vi "Test PC from CnfgFile.vi"() -> ()   [LabVIEW 2009, in "POLARIS BME DG.lvlib"]
doc: "This VI is a example for usage of POLARIS BME DG.lvlib classes.\n\nUSAGE:\n1. Select Your .bmedg configiration file, with has been created with Configure Systems.vi\n2. Select directory that contains calibration filesl Modules.cal and BME_G0x.cal\n3. Enter the name of the system whose channels Your want to modify\n4. Run VI\n5. Update Chnl Direct writes channel settings into HW with immediately deactivation, modify and activation of all system DGs. This will cause a common shot at all channels after activation. Please keep it in mind, if Your plant needs some pause between tho following shots e.g. for cool down.\n\n6. UpdateChnl synchron use mechanism of DG type SG08P2. You need to configure cards and channels properly for this reasen. All cards must have the same MS-Bus configuration and Bit \"LoadDataOnBus = 0x80\" mus be set. If all output modulo couner reach zero at MASTERCARD, mastercard puts a signal to slavecard to load new parameters.\n\n7. \"Update Chnl wait\" can be used if channels have slow repetition rate compared with polling rate of ReadTriggerCounter. Programm wait close before next common shot would fall and updates parameter with de and reactivate of all cards.\n\nIMPLEMENTATION: See comments in blockdiagramm.\n\n\n-----------------\n\nauthor: Alexander Kessler, Helmholtz-Institut-Jena \nmaintainer: Alexander Kessler: alexander.kessler@uni-jena.de\n\nLicense Agreement for this software:\n\nCopyright (C)\nHelmholtz-Institut-Jena\nFröbelsteg 3\n07743 Jena\nGermany\n\nContact: alexander.kessler@uni-jena.de\n\nThis program is free software; you can redistribute it and/or modify it under the terms of the GNU General Public License as published by the Free Software Foundation; either version 2 of the license, or (at your option) any later version.\n\nThis program is distributed in the hope that it will be useful, but WITHOUT ANY WARRANTY; without even the implied warranty of MERCHANTABILITY or FITNESS FOR A PARTICULAR PURPOSE. See the GNU General License for more details (http://www.gnu.org)."
uses:
  POLARIS BME DG.lvlib
  LV-BME Interface/ChnlSettings.ctl
  LV-BME Interface/Chnl Settings Complete.ctl
  LV-BME Interface/Go_Done_Chnl_Settings.ctl
  LV-BME Interface/GoSignalBits.ctl
  LV-BME Interface/SG08_Chnl_Settings.ctl
  DG Classes/BME_DG_Chnl/BME_DG_Chnl.lvclass
  DG Classes/BME_DG_Base/BME_DG_Base.lvclass
  DG Classes/BME_DG_System/BME_DG_System.lvclass
panel:
  out "ChnlPeriods":dbl[][](array[numeric])
  in  "Save Changes":bool=TRUE
  out "Master Trigger Counter":i64
  in  "SystemlName":u16(ring) items=["MiraSync", "MS"]
  in  "UpdateChnl Synchron":bool=TRUE
  in  "ChnlParam":T1={"Channel Name"="", "ChnParameter"={" Delay (µs)"=0.0, "On?"=FALSE, "PositiveVoltage?"=TRUE, "50OhmTerminated? "=FALSE, "25OhmOutput?"=FALSE}, "DelayFormula"="", "OutputModulo"=1, "Go and Done Signal"={"Go Signal"=16, "Done Signal"=16}, "G08_Chnl_Settings"={"Pulse Width (µs)"=0.1, "Output Offset"=0, "Disconnect (E,F)"=FALSE, "Onto MsBus (E,F)"=FALSE, "Input Positive (E,F)"=TRUE}} {"ChnParameter"."Delay (µs)" min=0.0 max=100000000.0 format="%.4f"; "G08_Chnl_Settings"."Pulse Width (µs)" min=0.0 max=8947840.0 format="%#.6f"; "Go and Done Signal"."Done Signal" format="%04x" items=["Local Primary"=1, "Local Secondary"=2, "Local Force"=4, "Master Primary"=16]; "Go and Done Signal"."Go Signal" format="%04x" items=["Local Primary0x1"=1, "Local Secondary0x2"=2, "Local Force 0x4"=4, "Resynchronize 0x8"=8, "Master Prim. 0x10"=16, "Master Sec. 0x20"=32, "Master Force  0x40"=64, "System Clock 0x80"=128, "Delay Clock 0x100"=256, "Inhibit Local 0x200"=512, "Start Local 0x400"=1024, "Start Bus 0x800"=2048, "Step Back Local 0x1000"=4096, "Step Back Bus 0x2000"=8192, "RunCircle 0x4000"=16384, "SyncReload 0x8000"=32768, "From E 0x10000"=65536, "From F 0x20000"=131072, "From Bus 0x40000"=262144]}
  in  "Update Chnl direct":bool=TRUE
  in  "pathCalFilesDir":path=path "C:/CS Framework/pwpc74-Config"
  in  "pathConfigFile":path=path "C:/CS Framework/pwpc74-Config/pwpc74.bmedg"
  out "Problem Chnls out":string[](array[string])
  in  "Reset Error":bool
  out "error out":errorcluster
  in  "Update Delay direct":bool=TRUE
  in  "UpdateChnl wait":bool=TRUE
  in  "ChnlParameter":T6 {"ChnParam2write"."Delay (µs)" min=0.0 max=100000000.0 format="%.4f"}
  out "Counts till common shot":i32=2147483647
  out "Interrupts":u32[](array[numeric])=[11153, 10240, 10240, 10240, 11008, 11008, 10240, 10240, 10240] format="%b"
  in  "stop 2":bool=TRUE
  in  "ReadStatus":bool=TRUE
  in  "Activate Card":bool=TRUE
  in  "ResetModuloCounters":bool=TRUE
  in  "Selected Chnl":u16(ring) items=["TrigDelay", "A1LDD", "A3LDD", "A4LDD", "A5LDD", "Reserve", "PulsP On", "PulsP Off", "A1 PC On", "A1 PC Off", "Oszi", "Kamera"]
  in  "Card":u16(ring) items=["Master", "Slave1"]
  in  "STOP":bool
  # "ATTENTION, WORKS ONLY\nif a MASTER CHNL  is set to \nsync update!!! Otherwise undefined\nDelay states occur."
  # "Calls of DLL \nSet_G08_Delay\nhave no effect\nindependent of sync\nsettings\n201207-10\n\n201211-26 LoadCardParam\ncall is needed"
  # "Funktioniert nicht, das Problem liegt daran, dass ulong ReadInterruptStatus(long DG_Number) die Interruptbits nicht\nzuverlässig ausliest."
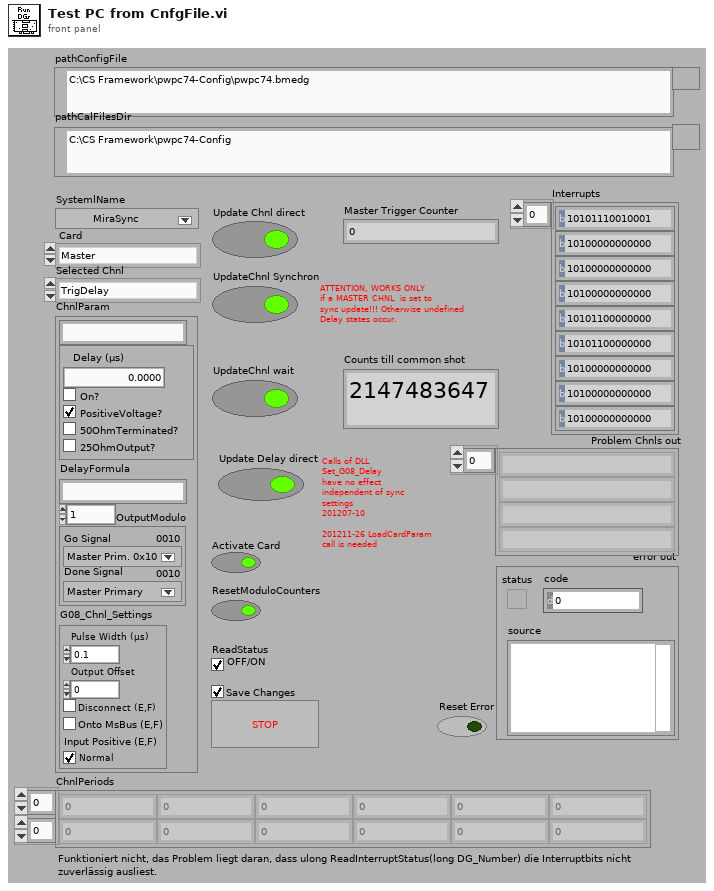
[diagram p1: front panel]
types:
  T1 = typedef "POLARIS BME DG.lvlib/Chnl Settings Complete.ctl" = cluster{"Channel Name":string, "ChnParameter":T2, "DelayFormula":string, "OutputModulo":i32, "Go and Done Signal":T3, "G08_Chnl_Settings":T5}
  T2 = typedef "POLARIS BME DG.lvlib/ChnlSettings.ctl" = cluster{" Delay (µs)":dbl, "On?":bool, "PositiveVoltage?":bool, "50OhmTerminated? ":bool, "25OhmOutput?":bool}
  T3 = typedef "POLARIS BME DG.lvlib/Go_Done_Chnl_Settings.ctl" = cluster{"Go Signal":T4, "Done Signal":u32}
  T4 = typedef "POLARIS BME DG.lvlib/GoSignalBits.ctl" = u32
  T5 = typedef "POLARIS BME DG.lvlib/SG08_Chnl_Settings.ctl" = cluster{"Pulse Width (µs)":dbl, "Output Offset":u32, "Disconnect (E,F)":bool, "Onto MsBus (E,F)":bool, "Input Positive (E,F)":bool}
  T6 = cluster{"ChnlName":string, "ChnParam2write":T2, "TriggerModulo":u32}
  T7 = enum16{"GetSystem", "SetSystem", "FirstInit", "ForceInit", "Release"}
  T8 = enum8{"Enabled", "Disabled", "Disabled and Grayed Out"}
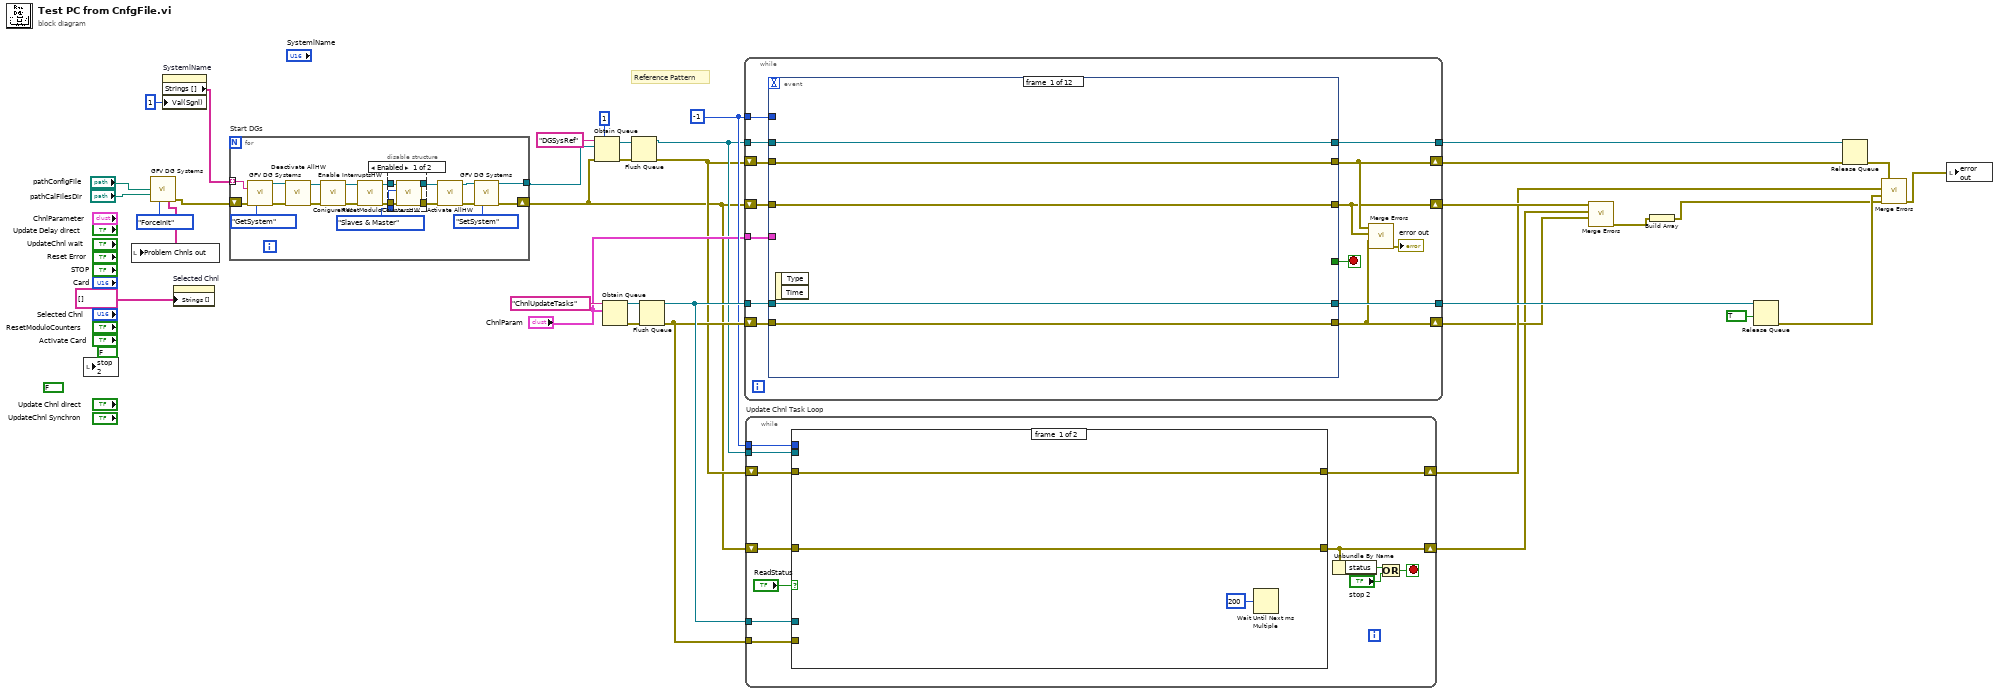
[diagram p0: block diagram]
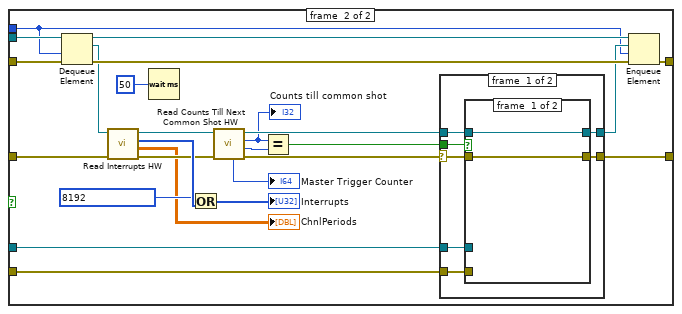
[diagram p3: hidden frame]
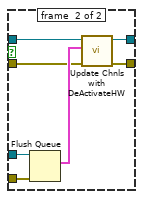
[diagram p4: hidden frame]
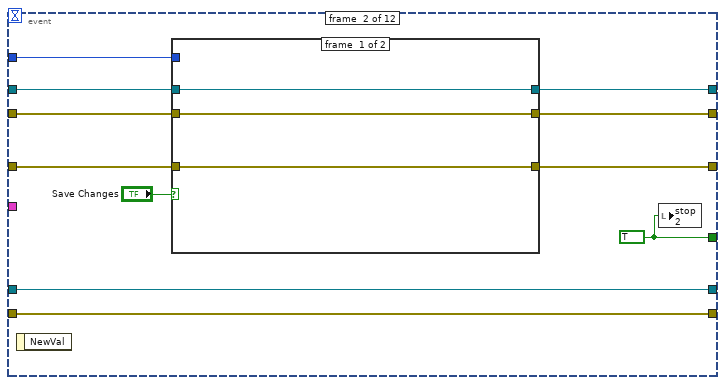
[diagram p6: hidden frame]
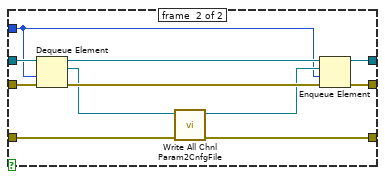
[diagram p7: hidden frame]
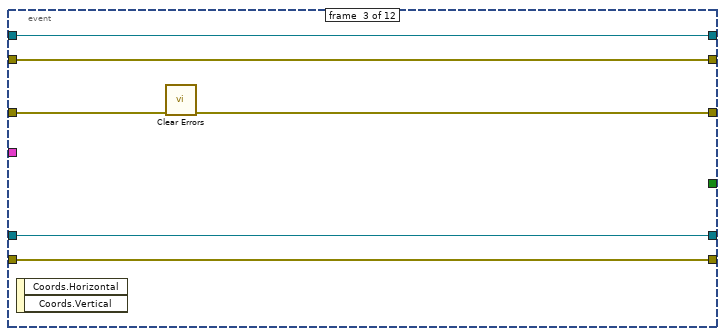
[diagram p8: hidden frame]
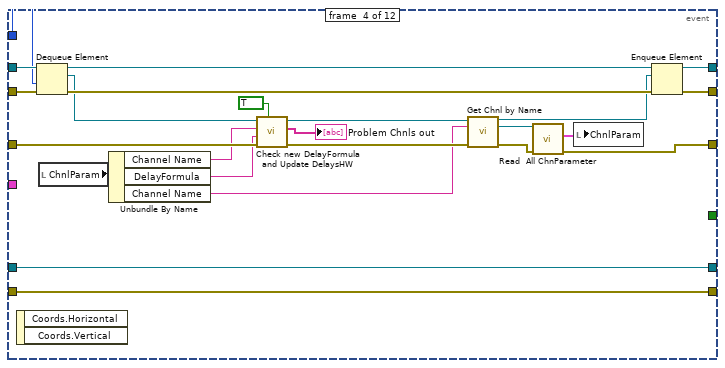
[diagram p9: hidden frame]
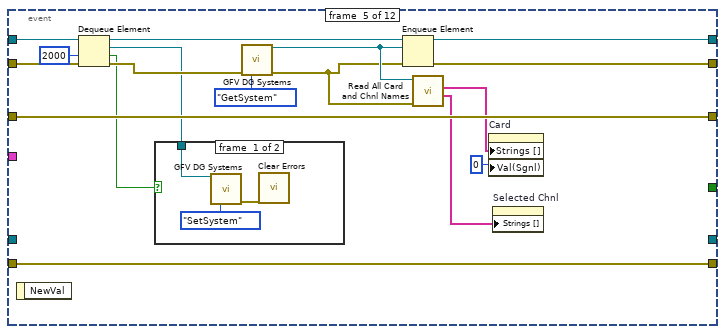
[diagram p10: hidden frame]
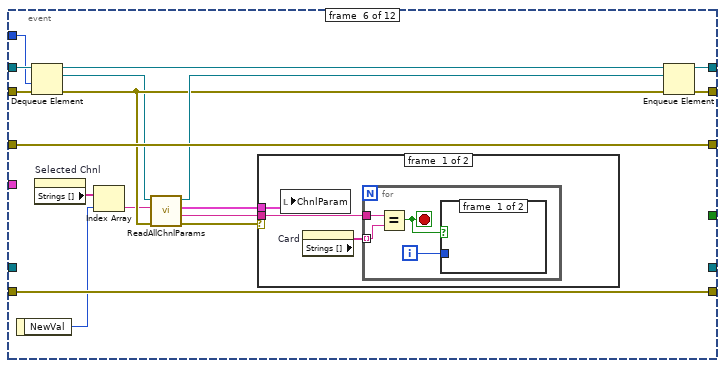
[diagram p12: hidden frame]
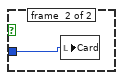
[diagram p13: hidden frame]
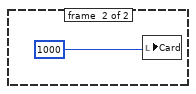
[diagram p14: hidden frame]
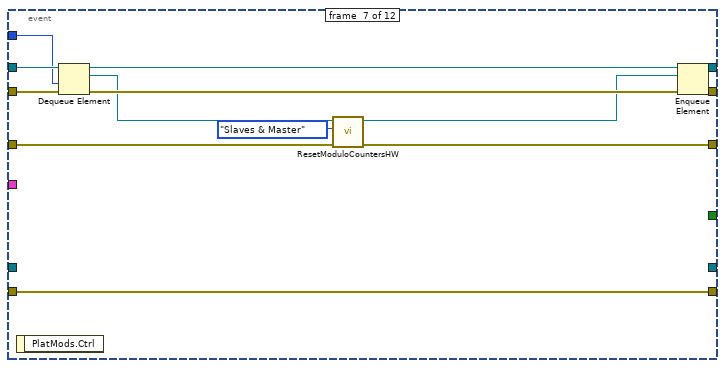
[diagram p15: hidden frame]
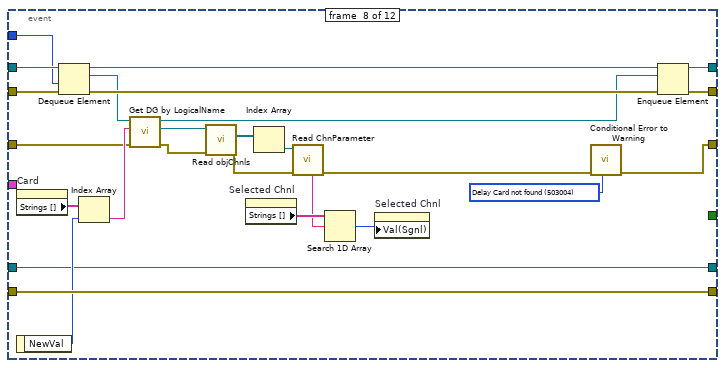
[diagram p16: hidden frame]
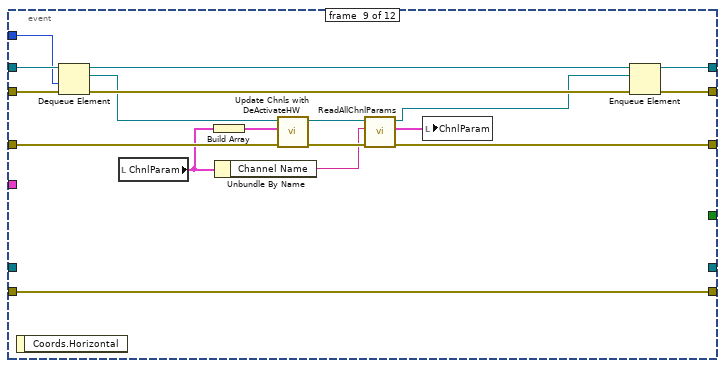
[diagram p17: hidden frame]
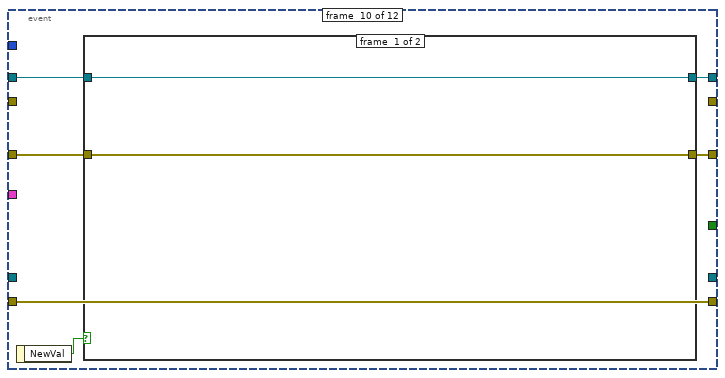
[diagram p18: hidden frame]
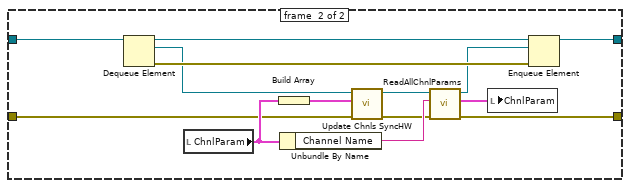
[diagram p19: hidden frame]
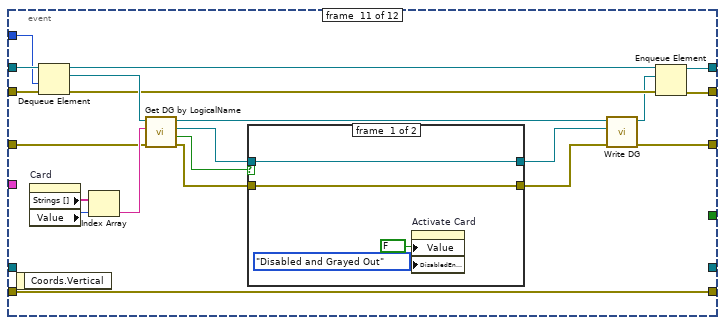
[diagram p20: hidden frame]
diagram:
  w23 = -1 ("timeout in ms (-1)")
  (unwired) FALSE ("stop 3")
  # "Reference Pattern"
  n1 = local write "stop 2"(FALSE ("stop 2")) -> ()
  n2 = call "GFV DG Systems.vi"("Config File"="pathConfigFile", "Dir Calibration files"="pathCalFilesDir", "Mode"=T7."ForceInit") -> ("Problem Chnls out"=w13:string[], "error out"=w14:errorcluster)  [unwired: 7 in, 4 out]
  n3 = local write "Problem Chnls out"(w13) -> ()
  n4 = property on="SystemlName" class="Ring (strict)"("Val(Sgnl)"=u16 1 ("Value (Signaling)")) -> ("Strings []"=w12:string[])  [unwired: 2 in, 2 out]
  n5 = property on="Selected Chnl" class="Ring (strict)"("Strings []"=string[] []) -> ()  [unwired: 2 in, 2 out]
  n6 = for "Start DGs" {
    shift-right: [w39] -> w8
    shift-left: w14 -> [w45]
    tunnel: w12 -> [w44] mode=indexing
    tunnel: [w38] -> w7
    n7 = call "GFV DG Systems.vi"("SystemlName"=w44, "error in"=w45, "Mode"=T7."GetSystem") -> ("BME_DG_System out"=w43:refnum<class "BME_DG_System.lvclass">, "error out"=w46:errorcluster)  [unwired: 7 in, 4 out]
    n8 = call "Deactivate AllHW.vi"("error in (no error)"=w46, "BME_DG_System in"=w43) -> ("error out"=w55:errorcluster, "BME_DG_System out"=w56:refnum<class "BME_DG_System.lvclass">)  [unwired: 8 in]
    n9 = call "ConigureHW.vi"("error in (no error)"=w55, "BME_DG_System in"=w56) -> ("error out"=w53:errorcluster, "BME_DG_System out"=w54:refnum<class "BME_DG_System.lvclass">)  [unwired: 8 in]
    n10 = call "Enable InterruptsHW.vi"("error in (no error)"=w53, "BME_DG_System in"=w54) -> ("error out"=w50:errorcluster, "BME_DG_System out"=w51:refnum<class "BME_DG_System.lvclass">)  [unwired: 8 in]
    n11 = disable-structure shown="Enabled" {
      disable-tunnel: w51 -> [w61 w63]
      disable-tunnel: [w60 w63] -> w49
      disable-tunnel: w50 -> [w59 w62]
      disable-tunnel: [w58 w62] -> w48
      disable-tunnel: enum16{"Slaves only", "Slaves & Master"}."Slaves & Master" ("Enum") -> [w57 _]
      frame #0 {
        n12 = call "ResetModuloCountersHW.vi"("error in (no error)"=w59, "Enum"=w57, "BME_DG_System in"=w61) -> ("error out"=w58:errorcluster, "BME_DG_System out"=w60:refnum<class "BME_DG_System.lvclass">)  [unwired: 7 in]
      }
      frame #1 {
      }
    }
    n13 = call "Activate AllHW.vi"("error in (no error)"=w48, "BME_DG_System in"=w49) -> ("error out"=w41:errorcluster, "BME_DG_System out"=w42:refnum<class "BME_DG_System.lvclass">)  [unwired: 8 in]
    n14 = call "GFV DG Systems.vi"("BME_DG_System"=w42, "error in"=w41, "Mode"=T7."SetSystem") -> ("BME_DG_System out"=w38:refnum<class "BME_DG_System.lvclass">, "error out"=w39:errorcluster)  [unwired: 7 in, 4 out]
  }
  n15 = Obtain Queue(max queue size (-1, unlimited)=1, name (unnamed)="DGSysRef", element data type=w7, error in (no error)=w8) -> (queue out=w33:refnum<queue>, error out=w32:errorcluster)  [unwired: 1 in, 1 out]
  n16 = Obtain Queue(name (unnamed)="ChnlUpdateTasks", element data type="ChnlParam") -> (queue out=w28:refnum<queue>, error out=w29:errorcluster)  [unwired: 3 in, 1 out]
  n17 = Flush Queue(queue=w33, error in (no error)=w32) -> (queue out=w10:refnum<queue>, error out=w9:errorcluster)  [unwired: 1 out]
  n18 = Flush Queue(queue=w28, error in (no error)=w29) -> (queue out=w25:refnum<queue>, error out=w24:errorcluster)  [unwired: 1 out]
  n19 = while {
    shift-right: [w66] -> w21
    shift-left: w8 -> [w75]
    shift-right: [w67] -> w6
    shift-left: w9 -> [w73]
    tunnel: w10 -> [w76]
    tunnel: [w74] -> w34
    tunnel: w25 -> [w72]
    tunnel: "ChnlParam" -> [w71]
    tunnel: [w69] -> w27
    shift-right: [w65] -> w19
    shift-left: w24 -> [w70]
    tunnel: w23 -> [w68]
    stop <- w77 stop-if-true
    n20 = event shown="[1] \"STOP\": Value Change" {
      selector: _ -> [_ _ _ _ _ _ _ _ _ _ _ _]
      dyn-events: _ -> [_ _ _ _ _ _ _ _ _ _ _ _]
      timeout: _ -> [_ _ _ _ _ _ _ _ _ _ _ _]
      tunnel: [_ w83 _ _ _ _ _ _ _ _ _ _] -> w77
      tunnel: w76 -> [w82 w90 w112 w136 w152 w169 w196 w222 w240 w244 w272 w312]
      tunnel: w75 -> [w81 w89 w113 w128 w154 w174 w186 w209 w232 w242 w280 w311]
      tunnel: [w82 w86 w112 w132 w149 w167 w191 w217 w235 w243 w266 w312] -> w74
      tunnel: [w81 w84 w108 w116 w154 w174 w187 w199 w226 w241 w273 w311] -> w66
      tunnel: w73 -> [w80 w88 w111 w135 w151 w168 w194 w220 w238 _ w271 w310]
      tunnel: [w80 w87 w111 w133 w148 w166 w192 w218 w236 _ w265 w310] -> w67
      tunnel: w72 -> [w79 w93 w110 w131 _ _ _ w201 _ _ _ w309]
      tunnel: w71 -> [_ _ _ _ _ _ _ _ _ _ _ _]
      tunnel: w70 -> [w78 w92 w109 w130 w153 w173 w190 w216 w234 w246 w264 w308]
      tunnel: [w79 w93 w110 w131 _ _ _ w201 _ _ _ w307] -> w69
      tunnel: [w78 w92 w109 w130 w153 w173 w190 w216 w234 w246 w264 w306] -> w65
      tunnel: w68 -> [_ w91 _ w123 _ w165 w184 w215 w233 _ w263 _]
      event #0 {
        n21 = event-data() -> ()  [unwired: 1 in, 2 out]
      }
      event #1 {
        w83 = TRUE
        n22 = event-data() -> ()  [unwired: 1 in, 1 out]
        n23 = case shown="True" "Save Changes" {
          tunnel: w90 -> [w94 w107]
          tunnel: w88 -> [w95 w105]
          tunnel: [w95 w103] -> w87
          tunnel: [w94 w102] -> w86
          tunnel: [w96 w99] -> w84
          tunnel: w89 -> [w96 w98]
          tunnel: w91 -> [_ w97]
          frame #0 {
          }
          frame #1 {
            n24 = Dequeue Element(queue=w107, timeout in ms (-1)=w97, error in (no error)=w105) -> (queue out=w106:refnum<queue>, element=w101:refnum<class "BME_DG_System.lvclass">, error out=w104:errorcluster)  [unwired: 1 out]
            n25 = call "Write All Chnl Param2CnfgFile.vi"("error in (no error)"=w98, "BME_DG_System in"=w101) -> ("error out"=w99:errorcluster, "BME_DG_System out"=w100:refnum<class "BME_DG_System.lvclass">)  [unwired: 8 in]
            n26 = Enqueue Element(queue=w106, element=w100, timeout in ms (-1)=w97, error in (no error)=w104) -> (queue out=w102:refnum<queue>, error out=w103:errorcluster)  [unwired: 1 out]
          }
        }
        n27 = local write "stop 2"(w83) -> ()
      }
      event #2 {
        n28 = event-data() -> ()  [unwired: 1 in, 2 out]
        n29 = call <vilib>:"Clear Errors.vi"("error in (no error)"=w113) -> ("error out"=w108:errorcluster)  [unwired: 6 in]
      }
      event #3 {
        n30 = event-data() -> ()  [unwired: 1 in, 2 out]
        n31 = Dequeue Element(queue=w136, timeout in ms (-1)=w123, error in (no error)=w135) -> (queue out=w137:refnum<queue>, element=w129:refnum<class "BME_DG_System.lvclass">, error out=w134:errorcluster)  [unwired: 1 out]
        n32 = local read "ChnlParam"() -> (w122:T1)
        n33 = Unbundle By Name(w122) -> ("Channel Name"=w119:string, "DelayFormula"=w121:string, "Channel Name"=w114:string)
        n34 = call "Check new DelayFormula and Update DelaysHW.vi"("Update HW?(false)"=TRUE ("Update HW"), "error in (no error)"=w128, "Delay Formula"=w121, "ChnlName"=w119, "BME_DG_System in"=w129) -> ("error out"=w125:errorcluster, "Problem Chnls out"=→"Problem Chnls out":string[], "BME_DG_System out"=w127:refnum<class "BME_DG_System.lvclass">)  [unwired: 3 in, 1 out]
        n35 = call "Get Chnl by Name.vi"("BME_DG_System in"=w127, "Chnl Name"=w114, "error in (no error)"=w125) -> ("BME_DG_System out"=w126:refnum<class "BME_DG_System.lvclass">, "BME_DG_Chnl"=w117:refnum<class "BME_DG_Chnl.lvclass">, "error out"=w118:errorcluster)  [unwired: 7 in, 3 out]
        n36 = call-dynamic "Read  All ChnParameter.vi"("error in (no error)"=w118, "BME_DG_Chnl in"=w117) -> ("error out"=w116:errorcluster, "ChnlParam"=w115:T1)  [unwired: 7 in, 1 out]
        n37 = local write "ChnlParam"(w115) -> ()
        n38 = Enqueue Element(queue=w137, element=w126, error in (no error)=w134) -> (queue out=w132:refnum<queue>, error out=w133:errorcluster)  [unwired: 1 in, 1 out]
      }
      event #4 {
        n39 = event-data() -> ()  [unwired: 1 in, 1 out]
        n40 = Dequeue Element(queue=w152, timeout in ms (-1)=2000, error in (no error)=w151) -> (queue out=w150:refnum<queue>, element=w140:refnum<class "BME_DG_System.lvclass">, timed out?=w138:bool, error out=w143:errorcluster)
        n41 = case shown="False" w138 {
          tunnel: w140 -> [w156 _]
          frame #0 {
            n42 = call "GFV DG Systems.vi"("BME_DG_System"=w156, "Mode"=T7."SetSystem") -> ("error out"=w155:errorcluster)  [unwired: 8 in, 5 out]
            n43 = call <vilib>:"Clear Errors.vi"("error in (no error)"=w155) -> ()  [unwired: 6 in, 1 out]
          }
          frame #1 {
          }
        }
        n44 = call "GFV DG Systems.vi"("error in"=w143, "Mode"=T7."GetSystem") -> ("BME_DG_System out"=w142:refnum<class "BME_DG_System.lvclass">, "error out"=w141:errorcluster)  [unwired: 8 in, 4 out]
        n45 = Enqueue Element(queue=w150, element=w142, error in (no error)=w141) -> (queue out=w149:refnum<queue>, error out=w148:errorcluster)  [unwired: 1 in, 1 out]
        n46 = call "Read All Card and Chnl Names.vi"("error in (no error)"=w141, "BME_DG_System in"=w142) -> ("ChnlNames"=w147:string[], "CardNames"=w146:string[])  [unwired: 6 in, 2 out]
        n47 = property on="Card" class="Ring (strict)"("Strings []"=w146, "Val(Sgnl)"=u16 0 ("Value (Signaling)")) -> ()  [unwired: 2 in, 2 out]
        n48 = property on="Selected Chnl" class="Ring (strict)"("Strings []"=w147) -> ()  [unwired: 2 in, 2 out]
      }
      event #5 {
        n49 = event-data() -> ("NewVal"=w171:u16)  [unwired: 1 in]
        n50 = Dequeue Element(queue=w169, timeout in ms (-1)=w165, error in (no error)=w168) -> (queue out=w170:refnum<queue>, element=w161:refnum<class "BME_DG_System.lvclass">, error out=w163:errorcluster)  [unwired: 1 out]
        n51 = property on="Selected Chnl" class="Ring (strict)"() -> ("Strings []"=w172:string[])  [unwired: 2 in, 2 out]
        n52 = Index Array(array=w172, index=w171) -> (element=w162:string)
        n53 = call "ReadAllChnlParams.vi"("error in (no error)"=w163, "ChnlName"=w162, "BME_DG_System in"=w161) -> ("error out"=w160:errorcluster, "Name of Card"=w159:string, "ChnlParam"=w158:T1, "BME_DG_System out"=w164:refnum<class "BME_DG_System.lvclass">)  [unwired: 5 in]
        n54 = case shown="No Error" w160 {
          tunnel: w159 -> [w176 _]
          tunnel: w158 -> [w175 _]
          frame #0 {
            n55 = local write "ChnlParam"(w175) -> ()
            n56 = property on="Card" class="Ring (strict)"() -> ("Strings []"=w177:string[])  [unwired: 2 in, 2 out]
            n57 = for {
              tunnel: w177 -> [w181] mode=indexing
              tunnel: w176 -> [w180]
              i -> [w178]
              stop <- w179 stop-if-true
              n58 = Equal?(x=w180, y=w181) -> (x = y?=w179:bool)
              n59 = case shown="True" w179 {
                tunnel: w178 -> [_ w182]
                frame #0 {
                }
                frame #1 {
                  n60 = local write "Card"(w182) -> ()
                }
              }
            }
          }
          frame #1 {
            n61 = local write "Card"(u16 1000 ("Value (Signaling)")) -> ()
          }
        }
        n62 = Enqueue Element(queue=w170, element=w164, error in (no error)=w163) -> (queue out=w167:refnum<queue>, error out=w166:errorcluster)  [unwired: 1 in, 1 out]
      }
      event #6 {
        n63 = event-data() -> ()  [unwired: 1 in, 1 out]
        n64 = Dequeue Element(queue=w196, timeout in ms (-1)=w184, error in (no error)=w194) -> (queue out=w195:refnum<queue>, element=w189:refnum<class "BME_DG_System.lvclass">, error out=w193:errorcluster)  [unwired: 1 out]
        n65 = call "ResetModuloCountersHW.vi"("error in (no error)"=w186, "Enum"=enum16{"Slaves only", "Slaves & Master"}."Slaves & Master", "BME_DG_System in"=w189) -> ("error out"=w187:errorcluster, "BME_DG_System out"=w188:refnum<class "BME_DG_System.lvclass">)  [unwired: 7 in]
        n66 = Enqueue Element(queue=w195, element=w188, error in (no error)=w193) -> (queue out=w191:refnum<queue>, error out=w192:errorcluster)  [unwired: 1 in, 1 out]
      }
      event #7 {
        w198 = 503004 items=["Channel refers itself"=503001, "Deadloop"=503002, "Negative Delay"=503003, "Delay Card not found"=503004, "Channel not found"=503005, "Parse Error"=503006, "Not Supported"=503007, "Systen not found"=503008, "To much masters"=503009, "None master in Syterm"=503010] ("error")
        n67 = property on="Card" class="Ring (strict)"() -> ("Strings []"=w214:string[])  [unwired: 2 in, 2 out]
        n68 = event-data() -> ("NewVal"=w213:u16)  [unwired: 1 in]
        n69 = Dequeue Element(queue=w222, timeout in ms (-1)=w215, error in (no error)=w220) -> (queue out=w221:refnum<queue>, element=w211:refnum<class "BME_DG_System.lvclass">, error out=w219:errorcluster)  [unwired: 1 out]
        n70 = Index Array(array=w214, index=w213) -> (element=w212:string)
        n71 = call "Get DG by LogicalName.vi"("error in (no error)"=w209, "LogicalName"=w212, "BME_DG_System in"=w211) -> ("error out"=w207:errorcluster, "BME_DG_Base.lvclass"=w208:refnum<class "BME_DG_Base.lvclass">, "BME_DG_System out"=w210:refnum<class "BME_DG_System.lvclass">)  [unwired: 5 in, 1 out]
        n72 = call-dynamic "Read objChnls.vi"("error in (no error)"=w207, "BME_DG_Base in"=w208) -> ("error out"=w204:errorcluster, "objChnls"=w206:refnum<class "BME_DG_Chnl.lvclass">[])  [unwired: 6 in, 2 out]
        n73 = property on="Selected Chnl" class="Ring (strict)"() -> ("Strings []"=w203:string[])  [unwired: 2 in, 2 out]
        n74 = Index Array(array=w206) -> (element=w205:refnum<class "BME_DG_Chnl.lvclass">)  [unwired: 1 in]
        n75 = call-dynamic "Read ChnParameter.vi"("error in (no error)"=w204, "BME_DG_Chnl in"=w205) -> ("error out"=w200:errorcluster, "Name"=w202:string)  [unwired: 4 in, 4 out]
        n76 = Search 1D Array(1D array=w203, element=w202) -> (index of element=w197:i32)  [unwired: 1 in]
        n77 = property on="Selected Chnl" class="Ring (strict)"("Val(Sgnl)"=w197) -> ()  [unwired: 2 in, 2 out]
        n78 = call "Conditional Error to Warning.vi"("Error Code"=w198, "error in"=w200) -> ("error out"=w199:errorcluster)  [unwired: 9 in]
        n79 = Enqueue Element(queue=w221, element=w210, error in (no error)=w219) -> (queue out=w217:refnum<queue>, error out=w218:errorcluster)  [unwired: 1 in, 1 out]
      }
      event #8 {
        n80 = event-data() -> ()  [unwired: 1 in, 1 out]
        n81 = Dequeue Element(queue=w240, timeout in ms (-1)=w233, error in (no error)=w238) -> (queue out=w239:refnum<queue>, element=w231:refnum<class "BME_DG_System.lvclass">, error out=w237:errorcluster)  [unwired: 1 out]
        n82 = local read "ChnlParam"() -> (w225:T1)
        n83 = Build Array(w225) -> (w230:T1[])
        n84 = Unbundle By Name(w225) -> ("Channel Name"=w224:string)
        n85 = call "Update Chnls with DeActivateHW.vi"("error in (no error)"=w232, "ChnlSettings"=w230, "BME_DG_System in"=w231) -> ("error out"=w227:errorcluster, "BME_DG_System out"=w229:refnum<class "BME_DG_System.lvclass">)  [unwired: 6 in, 1 out]
        n86 = call "ReadAllChnlParams.vi"("error in (no error)"=w227, "ChnlName"=w224, "BME_DG_System in"=w229) -> ("error out"=w226:errorcluster, "ChnlParam"=w223:T1, "BME_DG_System out"=w228:refnum<class "BME_DG_System.lvclass">)  [unwired: 5 in, 1 out]
        n87 = local write "ChnlParam"(w223) -> ()
        n88 = Enqueue Element(queue=w239, element=w228, error in (no error)=w237) -> (queue out=w235:refnum<queue>, error out=w236:errorcluster)  [unwired: 1 in, 1 out]
      }
      event #9 {
        n89 = event-data() -> ("NewVal"=w245:bool)  [unwired: 1 in]
        n90 = case shown="True" w245 {
          tunnel: w244 -> [w248 w256]
          tunnel: [w248 w255] -> w243
          tunnel: w242 -> [w247 w250]
          tunnel: [w247 w254] -> w241
          frame #0 {
          }
          frame #1 {
            n91 = Dequeue Element(queue=w256) -> (queue out=w262:refnum<queue>, element=w253:refnum<class "BME_DG_System.lvclass">, error out=w261:errorcluster)  [unwired: 2 in, 1 out]
            n92 = local read "ChnlParam"() -> (w259:T1)
            n93 = Build Array(w259) -> (w251:T1[])
            n94 = Unbundle By Name(w259) -> ("Channel Name"=w258:string)
            n95 = call "Update Chnls SyncHW.vi"("error in (no error)"=w250, "ChnlSettings"=w251, "BME_DG_System in"=w253) -> ("error out"=w249:errorcluster, "BME_DG_System out"=w252:refnum<class "BME_DG_System.lvclass">)  [unwired: 6 in, 1 out]
            n96 = call "ReadAllChnlParams.vi"("error in (no error)"=w249, "ChnlName"=w258, "BME_DG_System in"=w252) -> ("error out"=w254:errorcluster, "ChnlParam"=w257:T1, "BME_DG_System out"=w260:refnum<class "BME_DG_System.lvclass">)  [unwired: 5 in, 1 out]
            n97 = local write "ChnlParam"(w257) -> ()
            n98 = Enqueue Element(queue=w262, element=w260, error in (no error)=w261) -> (queue out=w255:refnum<queue>)  [unwired: 1 in, 2 out]
          }
        }
      }
      event #10 {
        n99 = event-data() -> ()  [unwired: 1 in, 1 out]
        n100 = property on="Card" class="Ring (strict)"() -> ("Strings []"=w283:string[], "Value"=w282:u16)  [unwired: 2 in, 2 out]
        n101 = Dequeue Element(queue=w272, timeout in ms (-1)=w263, error in (no error)=w271) -> (queue out=w269:refnum<queue>, element=w270:refnum<class "BME_DG_System.lvclass">, error out=w268:errorcluster)  [unwired: 1 out]
        n102 = Index Array(array=w283, index=w282) -> (element=w281:string)
        n103 = call "Get DG by LogicalName.vi"("error in (no error)"=w280, "LogicalName"=w281, "BME_DG_System in"=w270) -> ("error out"=w278:errorcluster, "found?"=w274:bool, "BME_DG_Base.lvclass"=w279:refnum<class "BME_DG_Base.lvclass">, "BME_DG_System out"=w275:refnum<class "BME_DG_System.lvclass">)  [unwired: 5 in]
        n104 = case shown="True" w274 {
          tunnel: w279 -> [w287 w294]
          tunnel: w278 -> [w286 w292]
          tunnel: [w286 w296] -> w277
          tunnel: [w287 w295] -> w276
          frame #0 {
            n105 = property on="Activate Card" class="Bool (strict)"("Value"=FALSE ("Activate"), "DisabledEnum"=T8."Disabled and Grayed Out" ("Disabled")) -> ()  [unwired: 2 in, 2 out]
          }
          frame #1 {
            n106 = call-dynamic "Read IsActive.vi"("error in (no error)"=w292, "BME_DG_Base in"=w294) -> ("error out"=w291:errorcluster, "Active?"=w290:bool, "BME_DG_Base out"=w293:refnum<class "BME_DG_Base.lvclass">)  [unwired: 7 in]
            n107 = Not(x=w290) -> (.not. x?=w288:bool)
            n108 = case shown="True" w290 {
              tunnel: [w300 w302] -> w296
              tunnel: [w299 w303] -> w295
              tunnel: w293 -> [w298 w304]
              tunnel: w291 -> [w297 w301]
              frame #0 {
                n109 = call "ActivateHW.vi"("error in (no error)"=w297, "BME_DG_Base in"=w298) -> ("error out"=w300:errorcluster, "BME_DG_Base out"=w299:refnum<class "BME_DG_Base.lvclass">)  [unwired: 8 in]
              }
              frame #1 {
                n110 = call-dynamic "DeactivateHW.vi"("error in (no error)"=w301, "BME_DG_Base in"=w304) -> ("error out"=w302:errorcluster, "BME_DG_Base out"=w303:refnum<class "BME_DG_Base.lvclass">)  [unwired: 6 in, 2 out]
              }
            }
            n111 = property on="Activate Card" class="Bool (strict)"("Value"=w288, "DisabledEnum"=T8."Enabled" ("Disabled")) -> ()  [unwired: 2 in, 2 out]
          }
        }
        n112 = call "Write DG.vi"("error in (no error)"=w277, "BME_DG_Base"=w276, "BME_DG_System in"=w275) -> ("error out"=w273:errorcluster, "BME_DG_System out"=w267:refnum<class "BME_DG_System.lvclass">)  [unwired: 7 in]
        n113 = Enqueue Element(queue=w269, element=w267, error in (no error)=w268) -> (queue out=w266:refnum<queue>, error out=w265:errorcluster)  [unwired: 1 in, 1 out]
      }
      event #11 {
        n114 = event-data() -> ()  [unwired: 1 in, 1 out]
        n115 = local read "ChnlParam"() -> (w305:T1)
        n116 = Enqueue Element(queue=w309, element=w305, error in (no error)=w308) -> (queue out=w307:refnum<queue>, error out=w306:errorcluster)  [unwired: 1 in, 1 out]
      }
    }
    n117 = call <vilib>:"Merge Errors.vi"("error in 3 (no error)"=w65, "error in 2 (no error)"=w66, "error in 1 (no error)"=w67) -> ("error out"=→"error out":errorcluster)  [unwired: 4 in]
  }
  n118 = while "Update Chnl Task Loop" {
    tunnel: w10 -> [w321]
    shift-right: [w319] -> w20
    shift-left: w9 -> [w320]
    shift-right: [w316] -> w18
    shift-left: w8 -> [w318]
    tunnel: w25 -> [w315]
    tunnel: w24 -> [w314]
    tunnel: w23 -> [w313]
    stop <- w323 stop-if-true
    n119 = case shown="True" "ReadStatus" {
      tunnel: w321 -> [_ w350]
      tunnel: w320 -> [w326 w349]
      tunnel: [w326 w348] -> w319
      tunnel: w318 -> [w325 w346]
      tunnel: [w325 w342] -> w316
      tunnel: w315 -> [_ w344]
      tunnel: w314 -> [_ w343]
      tunnel: w313 -> [_ w337]
      frame #0 {
        n120 = Wait Until Next ms Multiple(millisecond multiple=u32 200) -> ()  [unwired: 1 out]
      }
      frame #1 {
        n121 = Dequeue Element(queue=w350, timeout in ms (-1)=w337, error in (no error)=w349) -> (queue out=w351:refnum<queue>, element=w347:refnum<class "BME_DG_System.lvclass">, error out=w352:errorcluster)  [unwired: 1 out]
        n122 = call "Read Interrupts HW.vi"("error in (no error)"=w346, "BME_DG_System in"=w347) -> ("error out"=w335:errorcluster, "ChnlPeriods"=→"ChnlPeriods":dbl[][], "Interrupts"=w345:u32[], "BME_DG_System out"=w336:refnum<class "BME_DG_System.lvclass">)  [unwired: 6 in]
        n123 = Wait (ms)(milliseconds to wait=u32 50 ("millisecond multiple")) -> ()  [unwired: 1 out]
        n124 = Or(x=u32 8192, y=w345) -> (x .or. y?=→"Interrupts":u32[])
        n125 = call "Read Counts Till Next Common Shot HW.vi"("error in (no error)"=w335, "BME_DG_System in"=w336) -> ("error out"=w333:errorcluster, "LC Multiple"=w328:i64, "CountsRemains"=w329:i64, "BME_DG_System out"=w334:refnum<class "BME_DG_System.lvclass">, "Master Trigger Counter"=→"Master Trigger Counter":i64)  [unwired: 4 in, 1 out]
        "Counts till common shot" <- w329
        n126 = Equal?(x=w329, y=w328) -> (x = y?=w340:bool)
        n127 = case shown="No Error" w333 {
          selector: w333 -> [w356 w369]
          tunnel: w344 -> [w359 _]
          tunnel: w343 -> [w358 _]
          tunnel: w334 -> [w357 w370]
          tunnel: [w355 w369] -> w342
          tunnel: [w354 w370] -> w341
          tunnel: w340 -> [w353 _]
          frame #0 {
            n128 = case shown="True" w353 {
              tunnel: w359 -> [_ w368]
              tunnel: w358 -> [_ w367]
              tunnel: w357 -> [w361 w366]
              tunnel: w356 -> [w360 w364]
              tunnel: [w360 w363] -> w355
              tunnel: [w361 w362] -> w354
              frame #0 {
              }
              frame #1 {
                n129 = Flush Queue(queue=w368, error in (no error)=w367) -> (remaining elements=w365:T1[])  [unwired: 2 out]
                n130 = call "Update Chnls with DeActivateHW.vi"("error in (no error)"=w364, "ChnlSettings"=w365, "BME_DG_System in"=w366) -> ("error out"=w363:errorcluster, "BME_DG_System out"=w362:refnum<class "BME_DG_System.lvclass">)  [unwired: 6 in, 1 out]
              }
            }
          }
          frame #1 {
          }
        }
        n131 = Enqueue Element(queue=w351, element=w341, timeout in ms (-1)=w337, error in (no error)=w352) -> (error out=w348:errorcluster)  [unwired: 2 out]
      }
    }
    n132 = Unbundle By Name(w316) -> ("status"=w322:bool)
    n133 = Or(x=w322, y="stop 2") -> (x .or. y?=w323:bool)
  }
  n134 = call <vilib>:"Merge Errors.vi"("error in 3 (no error)"=w19, "error in 2 (no error)"=w18, "error in 1 (no error)"=w21) -> ("error out"=w2:errorcluster)  [unwired: 4 in]
  n135 = Build Array(w2) -> (w1:errorcluster[])
  n136 = Release Queue(queue=w27, force destroy? (F)=TRUE) -> (error out=w4:errorcluster)  [unwired: 1 in, 2 out]
  n137 = Release Queue(queue=w34, error in (no error)=w6) -> (error out=w5:errorcluster)  [unwired: 1 in, 2 out]
  n138 = call <vilib>:"Merge Errors.vi"("error array in"=w1, "error in 3 (no error)"=w4, "error in 2 (no error)"=w20, "error in 1 (no error)"=w5) -> ("error out"=w3:errorcluster)  [unwired: 3 in]
  n139 = local write "error out"(w3) -> ()
